vi "ChapterTenFinalProject.vi"() -> ()   [LabVIEW 2010]
uses:
  <vilib>/Instr/_visa.llb/VISA Configure Serial Port (Instr).vi
  <vilib>/Utility/inputDevices.llb/closeJoystick.vi
  <vilib>/Utility/inputDevices.llb/joystickAcquire.vi
panel:
  out "Serial Read":string
  in  "device index":i32=4
  in  "stop":bool
  out "Write Data":string
  in  "VISA resource name":refnum<visa-resource-name>
  out "error out":errorcluster
  in  "error in (no error)":errorcluster
  in  "Write":bool
  # "NatBot Interface"
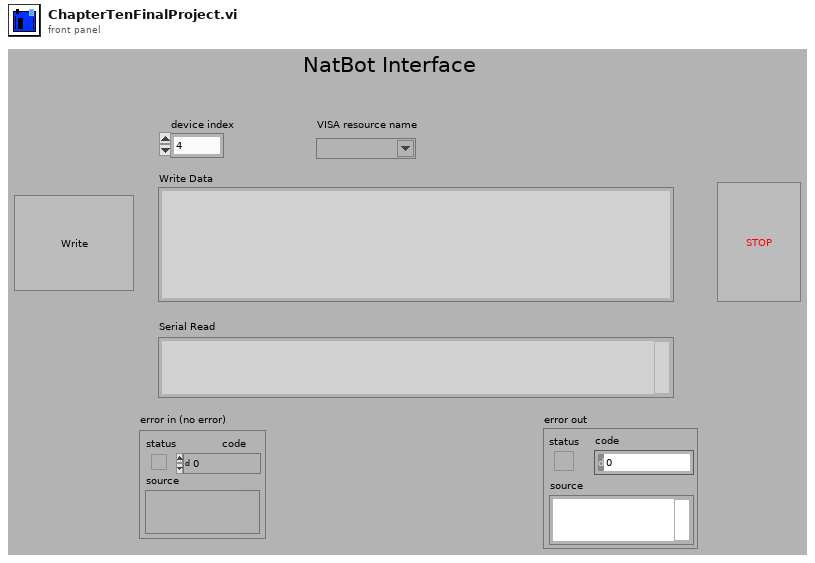
[diagram p1: front panel]
types:
  T1 = cluster{"X axis":i32, "Y axis":i32, "Z axis":i32, "X axis rotation":i32, "Y axis rotation":i32, "Z axis rotation":i32, "U axis":i32, "V axis":i32}
  T2 = cluster{"button 1":bool, "button 2":bool, "button 3":bool, "button 4":bool, "button 5":bool, "button 6":bool, "button 7":bool, "button 8":bool, "button 9":bool, "button 10":bool, "button 11":bool, "button 12":bool, "button 13":bool, "button 14":bool, "button 15":bool, "button 16":bool, "button 17":bool, "button 18":bool, "button 19":bool, "button 20":bool, "button 21":bool, "button 22":bool, "button 23":bool, "button 24":bool, "button 25":bool, "button 26":bool, "button 27":bool, "button 28":bool, "button 29":bool, "button 30":bool, "button 31":bool, "button 32":bool}
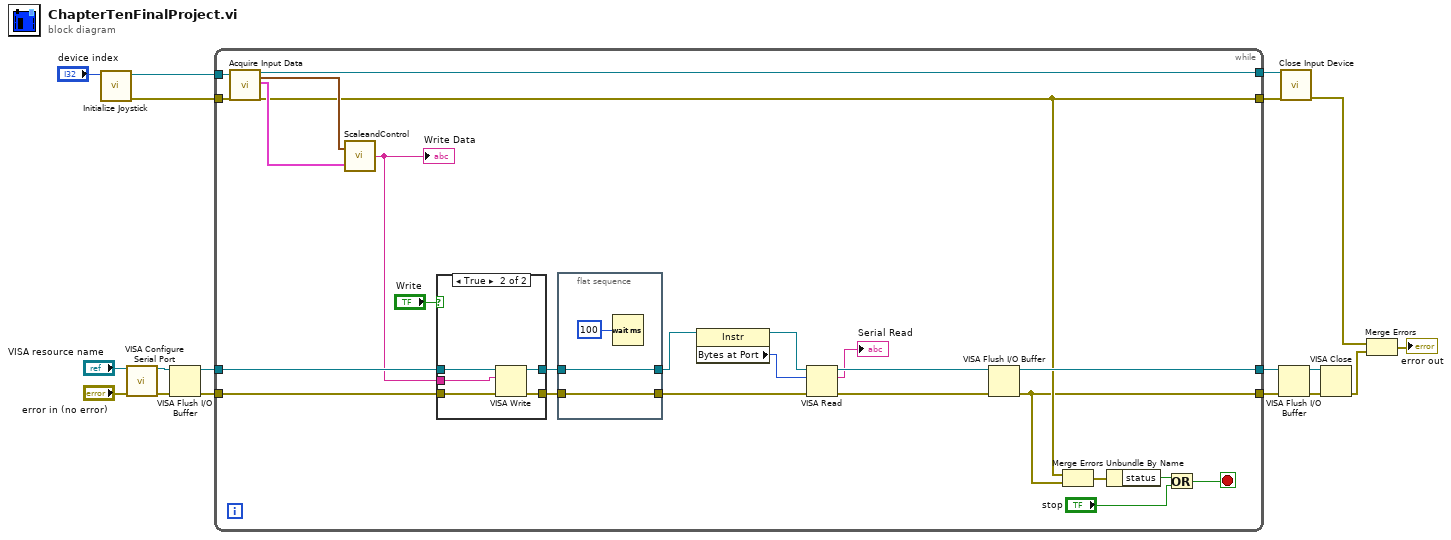
[diagram p0: block diagram]
diagram:
  n1 = call <vilib>:"Initialize Joystick.vi"("device index"="device index") -> ("error out"=w11:errorcluster, "device ID"=w12:refnum<k1>)  [unwired: 9 in]
  n2 = call-poly "VISA Configure Serial Port"("VISA resource name"="VISA resource name", "error in (no error)"="error in (no error)") -> ("VISA resource name out"=w13:refnum<visa-resource-name>, "error out"=w14:errorcluster)  [unwired: 12 in]
  n3 = VISA Flush I/O Buffer(VISA resource name=w13, error in (no error)=w14) -> (VISA resource name out=w8:refnum<visa-resource-name>, error out=w7:errorcluster)  [unwired: 1 in]
  n4 = while {
    tunnel: w12 -> [w42]
    tunnel: w11 -> [w41]
    tunnel: [w40] -> w10
    tunnel: [w27] -> w9
    tunnel: w8 -> [w33]
    tunnel: w7 -> [w32]
    tunnel: [w31] -> w6
    tunnel: [w26] -> w5
    stop <- w34 stop-if-true
    n5 = call-poly <vilib>:"Acquire Input Data.vi"("device ID"=w42, "error in (no error)"=w41) -> ("device ID"=w40:refnum<k1>, "axis info"=w43:T1, "button info"=w30:T2, "error out"=w27:errorcluster)  [unwired: 13 in, 1 out]
    n6 = call "ScaleandControl.vi"("button info"=w30, "axis info"=w43) -> ("String"=w29:string)
    "Write Data" <- w29
    n7 = case shown="True" "Write" {
      tunnel: [w48 w53] -> w38
      tunnel: [w47 w52] -> w39
      tunnel: w33 -> [w48 w51]
      tunnel: w32 -> [w47 w50]
      tunnel: w29 -> [_ w49]
      frame False {
      }
      frame True {
        n8 = VISA Write(VISA resource name=w51, write buffer=w49, error in (no error)=w50) -> (VISA resource name out=w53:refnum<visa-resource-name>, error out=w52:errorcluster)  [unwired: 1 out]
      }
    }
    n9 = flat-sequence {
      tunnel: w38 -> [w46]
      tunnel: [w46] -> w22
      tunnel: w39 -> [w45]
      tunnel: [w45] -> w25
      frame #0 {
        n10 = Wait (ms)(milliseconds to wait=u32 100) -> ()  [unwired: 1 out]
      }
    }
    n11 = property class="Instr"(reference=w22) -> (reference out=w21:refnum<visa-resource-name>, "Bytes at Port"=w20:u32)  [unwired: 1 in, 1 out]
    n12 = VISA Read(VISA resource name=w21, byte count=w20, error in (no error)=w25) -> (VISA resource name out=w24:refnum<visa-resource-name>, read buffer=→"Serial Read":string, error out=w23:errorcluster)  [unwired: 1 out]
    n13 = VISA Flush I/O Buffer(VISA resource name=w24, error in (no error)=w23) -> (VISA resource name out=w31:refnum<visa-resource-name>, error out=w26:errorcluster)  [unwired: 1 in]
    n14 = Merge Errors(w27, w26) -> (w28:errorcluster)
    n15 = Unbundle By Name(w28) -> ("status"=w37:bool)
    n16 = Or(x=w37, y="stop") -> (x .or. y?=w34:bool)
  }
  n17 = VISA Flush I/O Buffer(VISA resource name=w6, error in (no error)=w5) -> (VISA resource name out=w15:refnum<visa-resource-name>, error out=w16:errorcluster)  [unwired: 1 in]
  n18 = call-poly <vilib>:"Close Input Device.vi"("error in (no error)"=w9, "device ID"=w10) -> ("error out"=w1:errorcluster)  [unwired: 8 in]
  n19 = VISA Close(VISA resource name=w15, error in (no error)=w16) -> (error out=w3:errorcluster)
  n20 = Merge Errors(w1, w3) -> (→"error out":errorcluster)
